vi "ISO8601 DateString_new to Timestamp.vi"(9 "Strict ISO? (T)":bool=TRUE, 11 "ISO8601 DateString":string) -> (1 "valid?":bool, 2 "ISO Format":T1, 3 "Timestamp":timestamp)   [LabVIEW 2017]
uses:
  ISO8601 Date Formats.ctl
  <vilib>/Utility/miscctls.llb/LVDateTimeRec.ctl
  Timestamp to ISO8601 Day.vi
  isLeapYear (integer).vi
  <vilib>/Utility/error.llb/Trim Whitespace One-Sided.vi
  <vilib>/regexp/Match Regular Expression.xnode
  DateTime.ISO8601.lvclass
panel:
  # "This VI has an unfortunate name because\n\"ISO8601 DateString to Timestamp.vi\" is deprecated\nbecause of (formerly) confusing name."
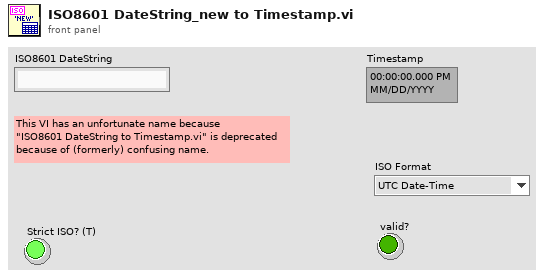
[diagram p1: front panel]
types:
  T1 = typedef "ISO8601 Date Formats.ctl" = enum16{"UTC Date-Time", "ISO Time", "Date", "Calendar Month", "Week", "Week-Day", "Month-Day", "Ordinal Date"}
  T2 = typedef "LVDateTimeRec.ctl" = cluster{"fractional second":dbl, "second":i32, "minute":i32, "hour":i32, "day of month":i32, "month":i32, "year":i32, "day of week":i32, "day of year":i32, "DST":i32}
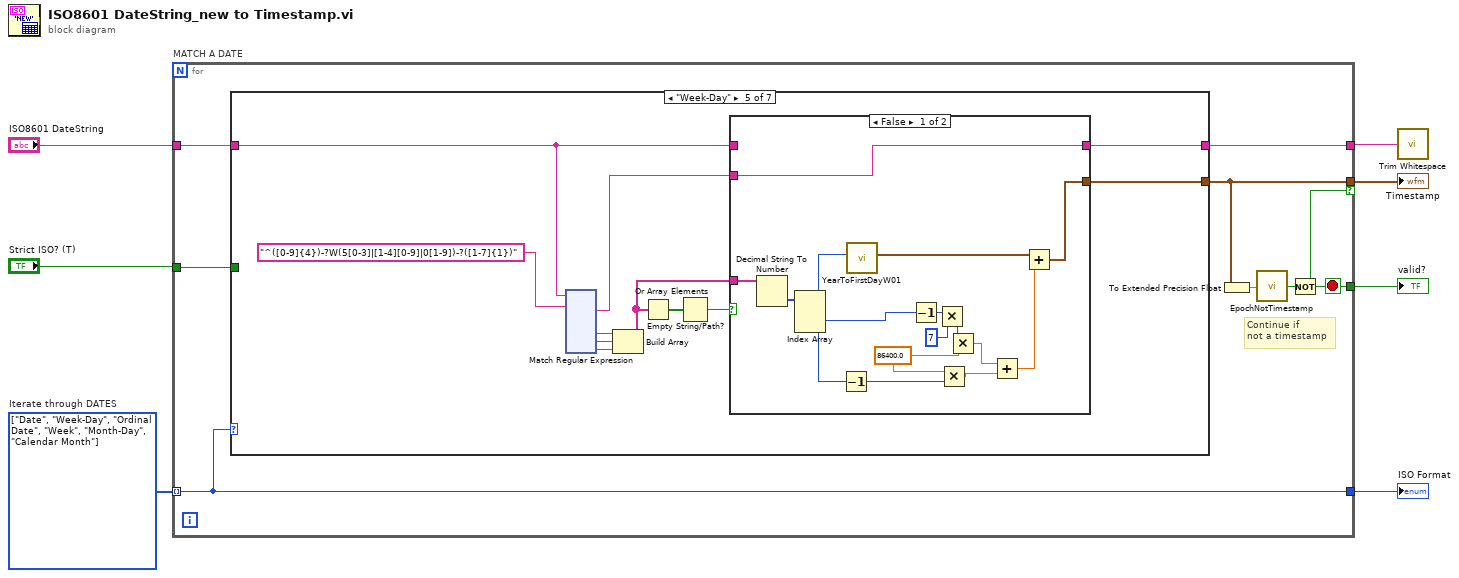
[diagram p0: block diagram]
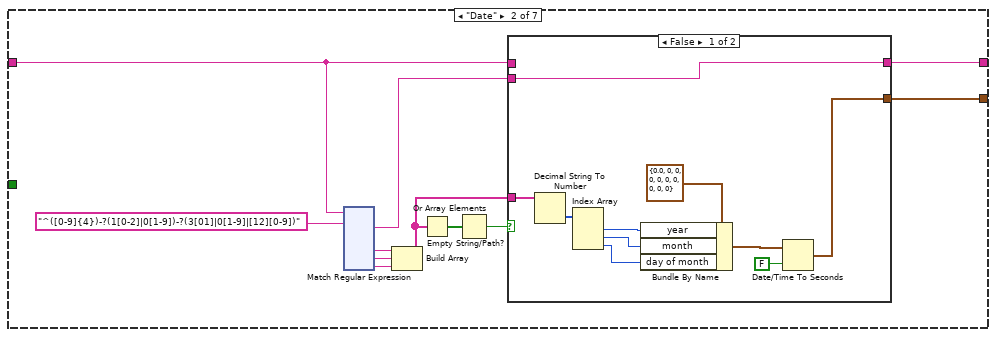
[diagram p3: hidden frame]
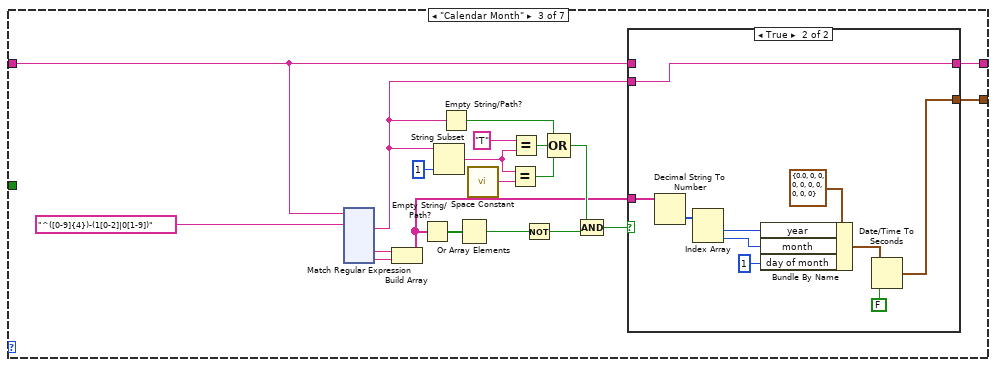
[diagram p5: hidden frame]
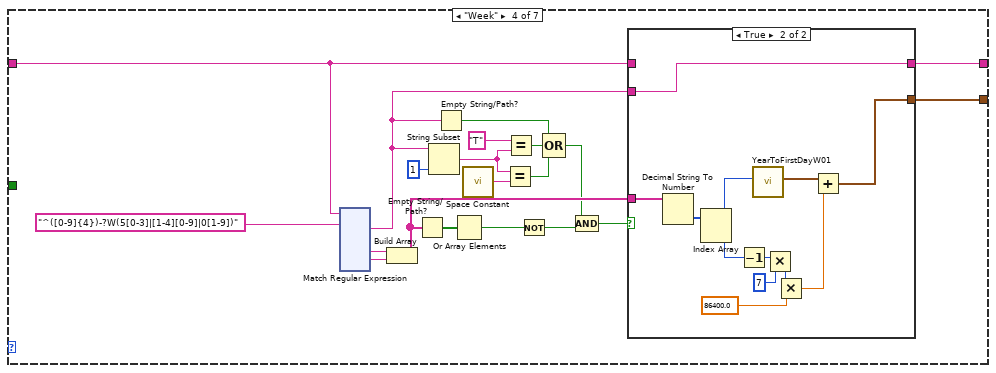
[diagram p7: hidden frame]
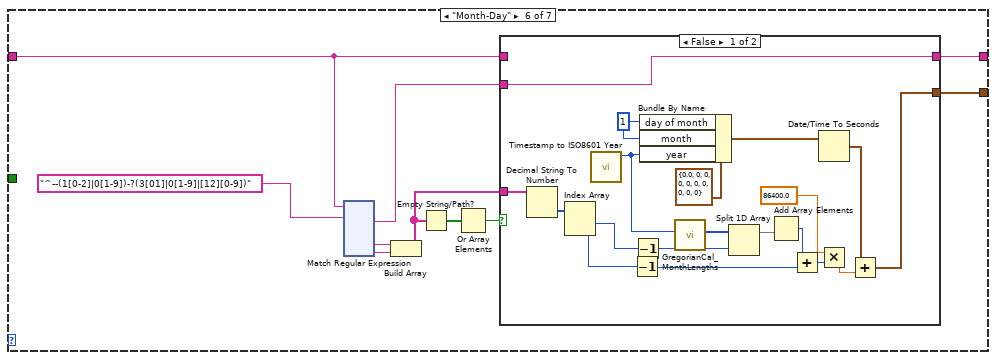
[diagram p10: hidden frame]
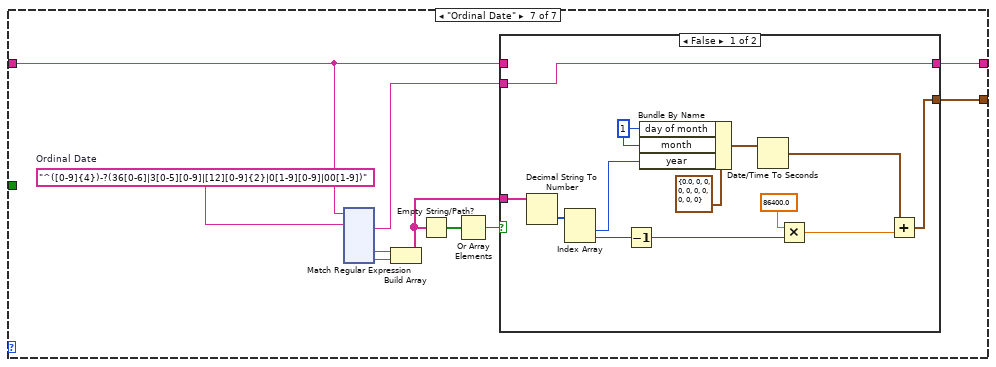
[diagram p12: hidden frame]
diagram:
  w1 = T1[] [enum."Date", enum."Week-Day", enum."Ordinal Date", enum."Week", enum."Month-Day", enum."Calendar Month"] items=["UTC Date-Time", "ISO Time", "Date", "Calendar Month", "Week", "Week-Day", "Month-Day", "Ordinal Date"]  # Iterate through DATES
  n1 = for "MATCH A DATE" {
    tunnel: "ISO8601 DateString" -> [w15]
    tunnel: [w8] -> w4
    tunnel: [w12] -> w5
    tunnel: w1 -> [w12] mode=indexing
    tunnel: "Strict ISO? (T)" -> [w11]
    tunnel: [w10] -> w2
    tunnel: [w9] -> w6 if=w8
    stop <- w8 stop-if-true
    # "Continue if\nnot a timestamp"
    n2 = case shown="\"Week-Day\"" w12 {
      tunnel: w15 -> [w16 w17 w160 w323 w466 w615 w764]
      tunnel: w11 -> [_ _ _ _ _ _ _]
      tunnel: [w16 w19 w178 w324 w467 w616 w766] -> w10
      tunnel: [_ w20 w179 w325 w469 w618 w767] -> w9
      frame Default {
        # "We process only DATES in this loop."
      }
      frame "Date" {
        n3 = xnode "Match Regular Expression"("input string"=w17, "regular expression"="^([0-9]{4})-?(1[0-2]|0[1-9])-?(3[01]|0[1-9]|[12][0-9])") -> ("after match"=w18:string, "submatch 1"=w27:string, "submatch 2"=w26:string, "submatch 3"=w25:string)  [unwired: 4 in, 4 out]
        n4 = Build Array(w27, w26, w25) -> (w21:string[])
        n5 = Empty String/Path?(string/path=w21) -> (empty?=w24:bool[])
        n6 = Or Array Elements(Boolean array=w24) -> (logical OR=w23:bool)
        n7 = case shown="False" w23 {
          tunnel: w21 -> [w157 _]
          tunnel: [w151 _] -> w20
          tunnel: [w150 w159] -> w19
          tunnel: w18 -> [w150 _]
          tunnel: w17 -> [_ w159]
          frame False {
            n8 = Decimal String To Number(string=w157) -> (number=w158:i32[])  [unwired: 2 in, 1 out]
            n9 = Index Array(array=w158) -> (element #1=w156:i32, element #2=w155:i32, element #3=w154:i32)  [unwired: 3 in]
            n10 = Bundle By Name(cluster=T2 {"fractional second"=0.0, "second"=0, "minute"=0, "hour"=0, "day of month"=0, "month"=0, "year"=0, "day of week"=0, "day of year"=0, "DST"=0} ("date time rec"), "year"=w156, "month"=w155, "day of month"=w154) -> (w153:T2)
            n11 = Date/Time To Seconds(1:FALSE ("is UTC (F)"), 2:w153) -> (0:w151:timestamp)
          }
          frame True {
          }
        }
      }
      frame "Calendar Month" {
        n12 = xnode "Match Regular Expression"("input string"=w160, "regular expression"="^([0-9]{4})-(1[0-2]|0[1-9])") -> ("after match"=w163:string, "submatch 1"=w164:string, "submatch 2"=w165:string)  [unwired: 4 in, 4 out]
        n13 = Build Array(w164, w165) -> (w162:string[])
        n14 = Empty String/Path?(string/path=w162) -> (empty?=w166:bool[])
        n15 = String Subset(string=w163, length (rest)=1 ("length (rest)")) -> (substring=w171:string)  [unwired: 1 in]
        n16 = Empty String/Path?(string/path=w163) -> (empty?=w167:bool)
        n17 = Or Array Elements(Boolean array=w166) -> (logical OR=w175:bool)
        n18 = call <vilib>:"Space Constant.vi"() -> ("String"=w173:string)
        n19 = Equal?(x=w171, y=w173) -> (x = y?=w172:bool)
        n20 = Equal?(x="T", y=w171) -> (x = y?=w170:bool)
        n21 = Not(x=w175) -> (.not. x?=w176:bool)
        n22 = Compound Arithmetic op=OR(w167, w170, w172) -> (w174:bool)
        n23 = Compound Arithmetic op=AND(w174, w176) -> (w161:bool)
        n24 = case shown="True" w161 {
          tunnel: w162 -> [_ w307]
          tunnel: [_ w302] -> w179
          tunnel: w160 -> [w300 _]
          tunnel: [w300 w301] -> w178
          tunnel: w163 -> [_ w301]
          frame False {
          }
          frame True {
            n25 = Decimal String To Number(string=w307) -> (number=w309:i32[])  [unwired: 2 in, 1 out]
            n26 = Index Array(array=w309) -> (element #1=w306:i32, element #2=w305:i32)  [unwired: 2 in]
            n27 = Bundle By Name(cluster=T2 {"fractional second"=0.0, "second"=0, "minute"=0, "hour"=0, "day of month"=0, "month"=0, "year"=0, "day of week"=0, "day of year"=0, "DST"=0} ("date time rec"), "year"=w306, "month"=w305, "day of month"=1) -> (w304:T2)
            n28 = Date/Time To Seconds(1:FALSE ("is UTC (F)"), 2:w304) -> (0:w302:timestamp)
          }
        }
      }
      frame "Week" {
        n29 = xnode "Match Regular Expression"("input string"=w323, "regular expression"="^([0-9]{4})-?W(5[0-3]|[1-4][0-9]|0[1-9])") -> ("after match"=w321:string, "submatch 1"=w330:string, "submatch 2"=w329:string)  [unwired: 4 in, 5 out]
        n30 = Build Array(w330, w329) -> (w326:string[])
        n31 = Empty String/Path?(string/path=w326) -> (empty?=w328:bool[])
        n32 = String Subset(string=w321, length (rest)=1 ("length (rest)")) -> (substring=w317:string)  [unwired: 1 in]
        n33 = Empty String/Path?(string/path=w321) -> (empty?=w322:bool)
        n34 = Or Array Elements(Boolean array=w328) -> (logical OR=w313:bool)
        n35 = call <vilib>:"Space Constant.vi"() -> ("String"=w315:string)
        n36 = Equal?(x=w317, y=w315) -> (x = y?=w316:bool)
        n37 = Equal?(x="T", y=w317) -> (x = y?=w318:bool)
        n38 = Not(x=w313) -> (.not. x?=w312:bool)
        n39 = Compound Arithmetic op=OR(w322, w318, w316) -> (w314:bool)
        n40 = Compound Arithmetic op=AND(w314, w312) -> (w311:bool)
        n41 = case shown="True" w311 {
          tunnel: w326 -> [_ w463]
          tunnel: [_ w454] -> w325
          tunnel: [w452 w453] -> w324
          tunnel: w321 -> [_ w453]
          tunnel: w323 -> [w452 _]
          frame False {
          }
          frame True {
            n42 = Decimal String To Number(string=w463) -> (number=w464:i32[])  [unwired: 2 in, 1 out]
            n43 = Index Array(array=w464) -> (element #1=w462:i32, element #2=w461:i32)  [unwired: 2 in]
            n44 = Decrement(x=w461) -> (x-1=w460:i32)
            n45 = call "YearToFirstDayW01.vi"("year"=w462) -> ("First Day of W01"=w456:timestamp)  [unwired: 10 in]
            n46 = Multiply(x=w460, y=7) -> (x*y=w459:i32)
            n47 = Multiply(x=w459, y=86400.0) -> (x*y=w455:dbl)
            n48 = Add(x=w456, y=w455) -> (x+y=w454:timestamp)
          }
        }
      }
      frame "Week-Day" {
        n49 = xnode "Match Regular Expression"("input string"=w466, "regular expression"="^([0-9]{4})-?W(5[0-3]|[1-4][0-9]|0[1-9])-?([1-7]{1})") -> ("after match"=w468:string, "submatch 1"=w475:string, "submatch 2"=w474:string, "submatch 3"=w470:string)  [unwired: 4 in, 4 out]
        n50 = Build Array(w475, w474, w470) -> (w471:string[])
        n51 = Empty String/Path?(string/path=w471) -> (empty?=w473:bool[])
        n52 = Or Array Elements(Boolean array=w473) -> (logical OR=w472:bool)
        n53 = case shown="False" w472 {
          tunnel: w471 -> [w611 _]
          tunnel: [w598 _] -> w469
          tunnel: [w597 w613] -> w467
          tunnel: w468 -> [w597 _]
          tunnel: w466 -> [_ w613]
          frame False {
            w601 = 86400.0
            n54 = Decimal String To Number(string=w611) -> (number=w612:i32[])  [unwired: 2 in, 1 out]
            n55 = Index Array(array=w612) -> (element #1=w610:i32, element #2=w609:i32, element #3=w602:i32)  [unwired: 3 in]
            n56 = Decrement(x=w602) -> (x-1=w600:i32)
            n57 = call "YearToFirstDayW01.vi"("year"=w610) -> ("First Day of W01"=w605:timestamp)  [unwired: 10 in]
            n58 = Decrement(x=w609) -> (x-1=w608:i32)
            n59 = Multiply(x=w608, y=7) -> (x*y=w607:i32)
            n60 = Multiply(x=w601, y=w600) -> (x*y=w599:dbl)
            n61 = Multiply(x=w607, y=w601) -> (x*y=w604:dbl)
            n62 = Add(x=w604, y=w599) -> (x+y=w603:dbl)
            n63 = Add(x=w605, y=w603) -> (x+y=w598:timestamp)
          }
          frame True {
          }
        }
      }
      frame "Month-Day" {
        n64 = xnode "Match Regular Expression"("input string"=w615, "regular expression"="^--(1[0-2]|0[1-9])-?(3[01]|0[1-9]|[12][0-9])") -> ("after match"=w617:string, "submatch 1"=w623:string, "submatch 2"=w622:string)  [unwired: 4 in, 4 out]
        n65 = Build Array(w623, w622) -> (w619:string[])
        n66 = Empty String/Path?(string/path=w619) -> (empty?=w621:bool[])
        n67 = Or Array Elements(Boolean array=w621) -> (logical OR=w620:bool)
        n68 = case shown="False" w620 {
          tunnel: w619 -> [w761 _]
          tunnel: [w745 _] -> w618
          tunnel: w617 -> [w744 _]
          tunnel: [w744 w763] -> w616
          tunnel: w615 -> [_ w763]
          frame False {
            w757 = 1 ("day of month")
            n69 = Decimal String To Number(string=w761) -> (number=w762:i32[])  [unwired: 2 in, 1 out]
            n70 = Index Array(array=w762) -> (element #1=w752:i32, element #2=w760:i32)  [unwired: 2 in]
            n71 = call "Timestamp to ISO8601 Year.vi"() -> ("year"=w754:i32)  [unwired: 10 in, 1 out]
            n72 = Decrement(x=w760) -> (x-1=w748:i32)
            n73 = Decrement(x=w752) -> (x-1=w751:i32)
            n74 = Bundle By Name(cluster=T2 {"fractional second"=0.0, "second"=0, "minute"=0, "hour"=0, "day of month"=0, "month"=0, "year"=0, "day of week"=0, "day of year"=0, "DST"=0} ("date time rec"), "day of month"=w757, "month"=w757, "year"=w754) -> (w758:T2)
            n75 = call "GregorianCal_MonthLengths.vi"("Year (0: this year)"=w754) -> ("Month Lengths"=w753:i32[])  [unwired: 10 in]
            n76 = Split 1D Array(array=w753, index=w751) -> (first subarray=w750:i32[])  [unwired: 1 out]
            n77 = Add Array Elements(numeric array=w750) -> (sum=w749:i32)
            n78 = Add(x=w749, y=w748) -> (x+y=w747:i32)
            n79 = Date/Time To Seconds(2:w758) -> (0:w755:timestamp)  [unwired: 1 in]
            n80 = Multiply(x=86400.0, y=w747) -> (x*y=w746:dbl)
            n81 = Add(x=w755, y=w746) -> (x+y=w745:timestamp)
          }
          frame True {
          }
        }
      }
      frame "Ordinal Date" {
        w768 = "^([0-9]{4})-?(36[0-6]|3[0-5][0-9]|[12][0-9]{2}|0[1-9][0-9]|00[1-9])"  # Ordinal Date
        n82 = xnode "Match Regular Expression"("input string"=w764, "regular expression"=w768) -> ("after match"=w765:string, "submatch 1"=w773:string, "submatch 2"=w772:string)  [unwired: 4 in, 4 out]
        n83 = Build Array(w773, w772) -> (w769:string[])
        n84 = Empty String/Path?(string/path=w769) -> (empty?=w771:bool[])
        n85 = Or Array Elements(Boolean array=w771) -> (logical OR=w770:bool)
        n86 = case shown="False" w770 {
          tunnel: w769 -> [w905 _]
          tunnel: [w895 _] -> w767
          tunnel: [w894 w907] -> w766
          tunnel: w765 -> [w894 _]
          tunnel: w764 -> [_ w907]
          frame False {
            w901 = 1 ("day of month")
            n87 = Decimal String To Number(string=w905) -> (number=w906:i32[])  [unwired: 2 in, 1 out]
            n88 = Index Array(array=w906) -> (element #1=w898:i32, element #2=w904:i32)  [unwired: 2 in]
            n89 = Decrement(x=w904) -> (x-1=w897:i32)
            n90 = Bundle By Name(cluster=T2 {"fractional second"=0.0, "second"=0, "minute"=0, "hour"=0, "day of month"=0, "month"=0, "year"=0, "day of week"=0, "day of year"=0, "DST"=0} ("date time rec"), "day of month"=w901, "month"=w901, "year"=w898) -> (w902:T2)
            n91 = Date/Time To Seconds(2:w902) -> (0:w896:timestamp)  [unwired: 1 in]
            n92 = Multiply(x=86400.0, y=w897) -> (x*y=w899:dbl)
            n93 = Add(x=w896, y=w899) -> (x+y=w895:timestamp)
          }
          frame True {
          }
        }
      }
    }
    n94 = To Extended Precision Float(1:w9) -> (0:w14:ext)
    n95 = call "EpochNotTimestamp.vi"("Epoch Time"=w14) -> ("Not a Timestamp?"=w13:bool)  [unwired: 8 in]
    n96 = Not(x=w13) -> (.not. x?=w8:bool)
  }
  "Timestamp" <- w6
  "ISO Format" <- w5
  "valid?" <- w4
  n97 = call <vilib>:"Trim Whitespace.vi"("string"=w2) -> ()  [unwired: 1 in, 1 out]
